vi "Set Conversion Table.vi"(8 "error in (no error)":errorcluster, 9 "Stepper":u32=1, 10 "Conversion table":dbl[][](array[numeric])=array38001x2[76002 elements], 11 "Stepper3D in":refnum<class "Stepper3D.lvclass">) -> (0 "error out":errorcluster, 3 "Stepper3D out":refnum<class "Stepper3D.lvclass">)   [LabVIEW 2014, in "Stepper3D.lvclass"]
uses:
  Stepper3D.lvclass
  Stepper3D.lvclass/Stepper3D.ctl
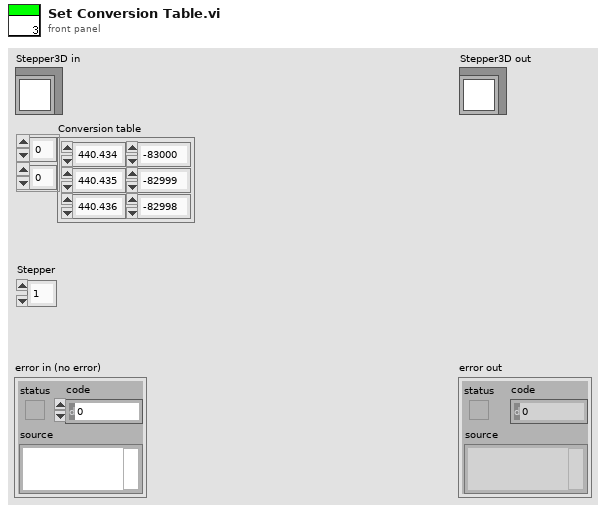
[diagram p1: front panel]
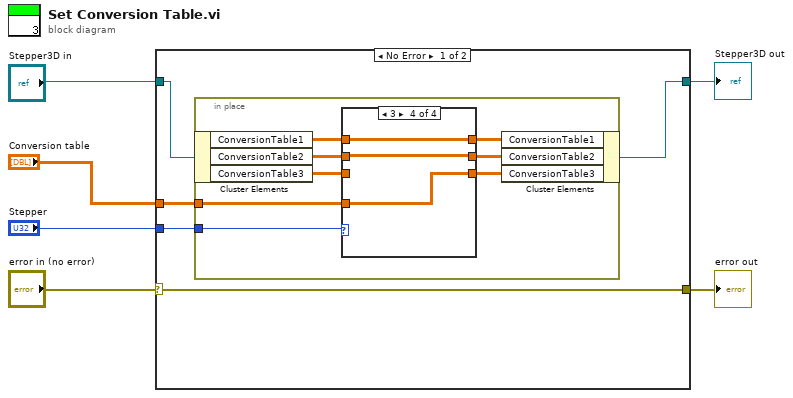
[diagram p0: block diagram]
diagram:
  n1 = case shown="No Error" "error in (no error)" {
    selector: "error in (no error)" -> [w11 w33]
    tunnel: [w11 w33] -> w5
    tunnel: [w8 w32] -> w1
    tunnel: "Stepper3D in" -> [w10 w32]
    tunnel: "Stepper" -> [w9 _]
    tunnel: "Conversion table" -> [w7 _]
    frame No Error {
      n2 = in-place {
        in-place-border: w9 -> [w19]
        in-place-border: w7 -> [w12]
        n3 = in-place-cluster #1(w10) -> ("ConversionTable1"=w17:dbl[][], "ConversionTable2"=w16:dbl[][], "ConversionTable3"=w13:dbl[][])
        n4 = case shown="3" w19 {
          tunnel: [w22 w25 w26 w31] -> w18
          tunnel: w17 -> [w22 _ w26 w31]
          tunnel: w16 -> [w21 w24 _ w30]
          tunnel: [w21 w24 w27 w30] -> w15
          tunnel: [w20 w23 w28 w29] -> w14
          tunnel: w13 -> [w20 w23 w28 _]
          tunnel: w12 -> [_ w25 w27 w29]
          frame Default {
          }
          frame 1 {
          }
          frame 2 {
          }
          frame 3 {
          }
        }
        n5 = in-place-cluster #1("ConversionTable1"=w18, "ConversionTable2"=w15, "ConversionTable3"=w14) -> (w8:refnum<class "Stepper3D.lvclass">)
      }
    }
    frame Error {
    }
  }
  "error out" <- w5
  "Stepper3D out" <- w1
